vi "InputPad.vi"(10 "Increments":enum32{"0.01", "0.1", "1", "10"}(radio), 11 "Num in":sgl) -> (3 "Num out":dbl format="%6.2f")   [LabVIEW 2012, in "StimulCtrls.lvlib"]
doc: "This VI is to create a two-digit number for cohort/electrode properties, including\n1. Frequency\n2. Pulse Width\n3. Signal Amplitude"
uses:
  StimulCtrls.lvlib
  UserControl/PadEnum.ctl
panel:
  in  "Enter":bool
  in  "Backspace":bool
  in  "Clear":bool
  in  "Up":bool
  in  "Down":bool
  in  "Dot":bool
  in  "NUM 9":bool
  in  "NUM 8":bool
  in  "NUM 7":bool
  in  "NUM 6":bool
  in  "NUM 5":bool
  in  "NUM 4":bool
  in  "NUM 3":bool
  in  "NUM 2":bool
  in  "NUM 1":bool
  in  "NUM 0":bool
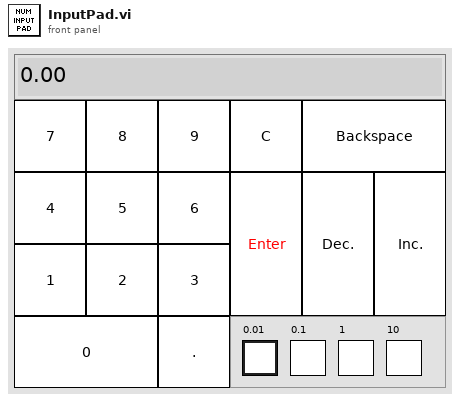
[diagram p1: front panel]
types:
  T1 = typedef "StimulCtrls.lvlib/PadEnum.ctl" = enum16{"Clear", "Inc/Dec", "Decrease", "Wait", "Exit", "Backspace", "InputDigit"}
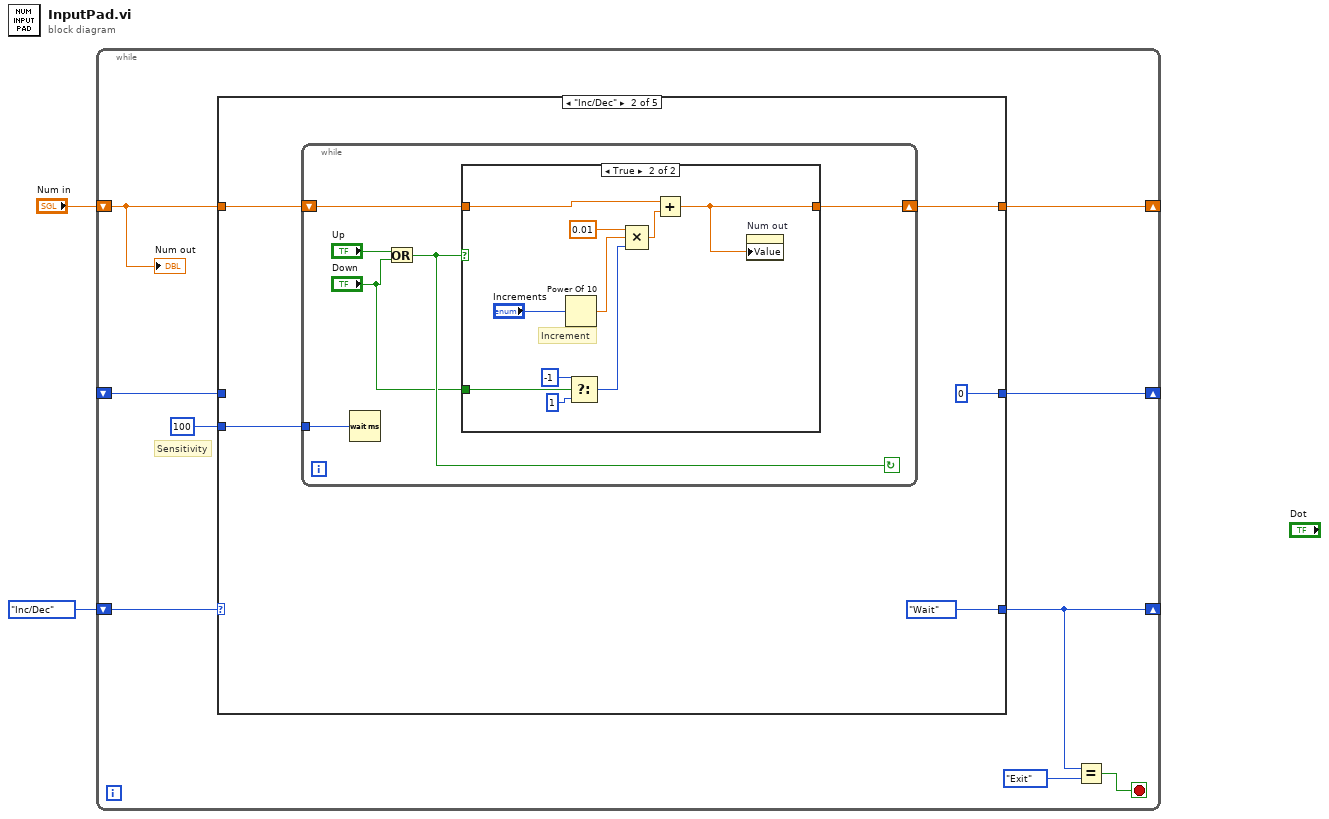
[diagram p0: block diagram]
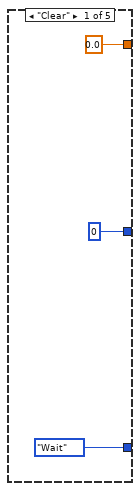
[diagram p2: hidden frame]
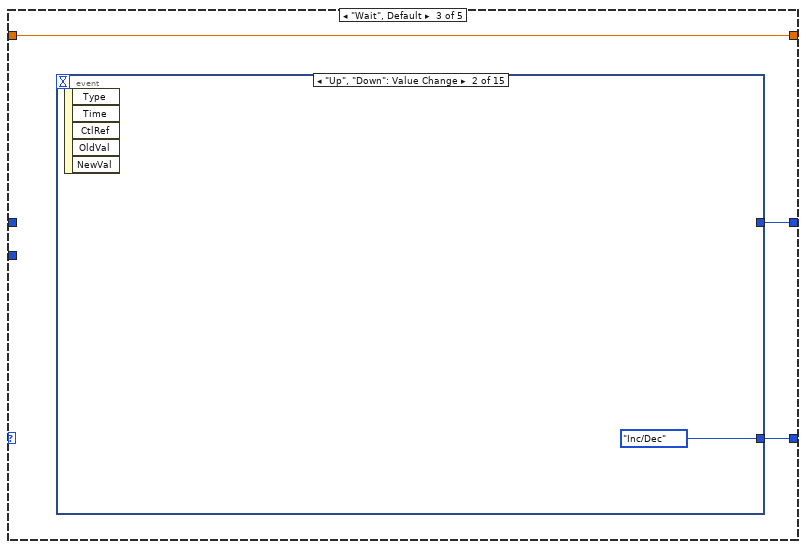
[diagram p4: hidden frame]
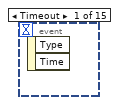
[diagram p5: hidden frame]
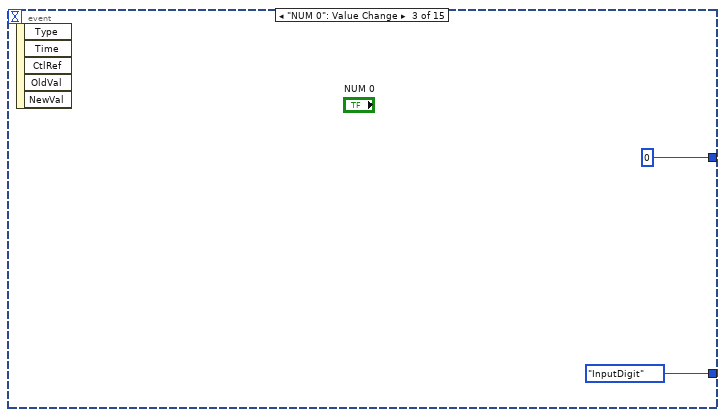
[diagram p6: hidden frame]
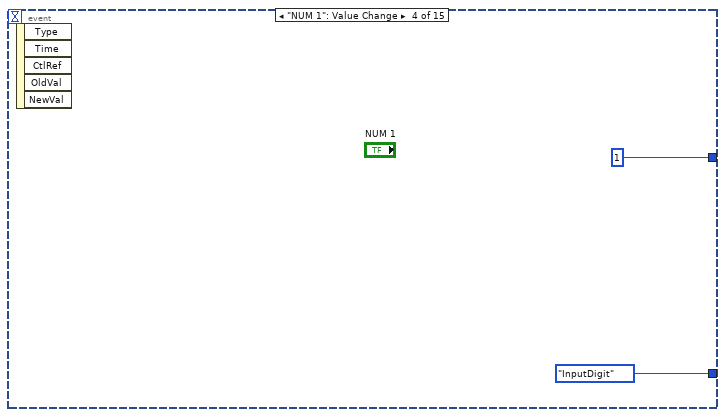
[diagram p7: hidden frame]
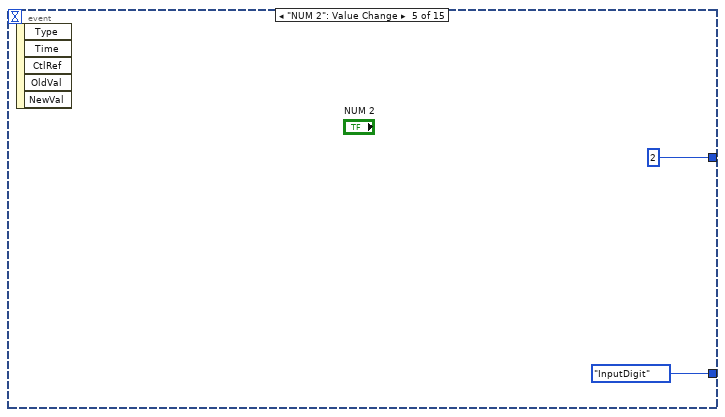
[diagram p8: hidden frame]
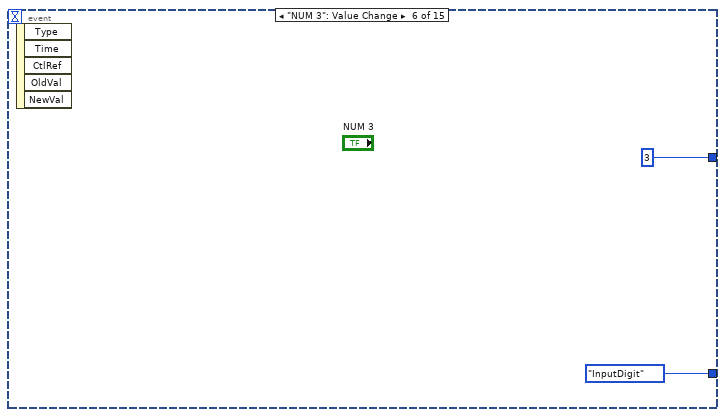
[diagram p9: hidden frame]
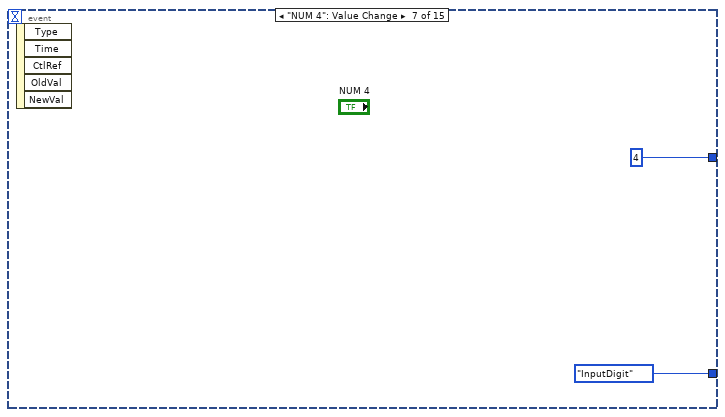
[diagram p10: hidden frame]
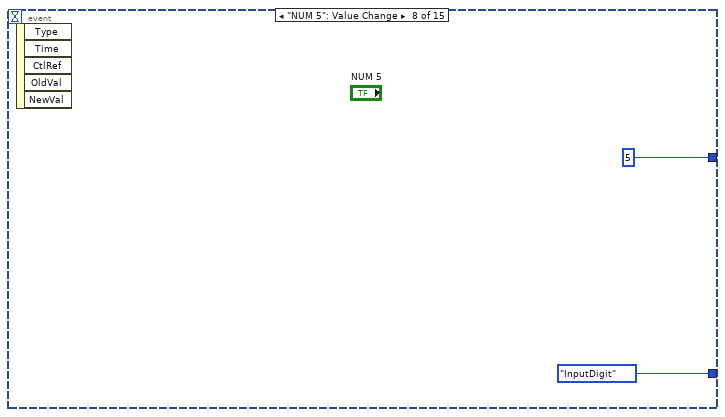
[diagram p11: hidden frame]
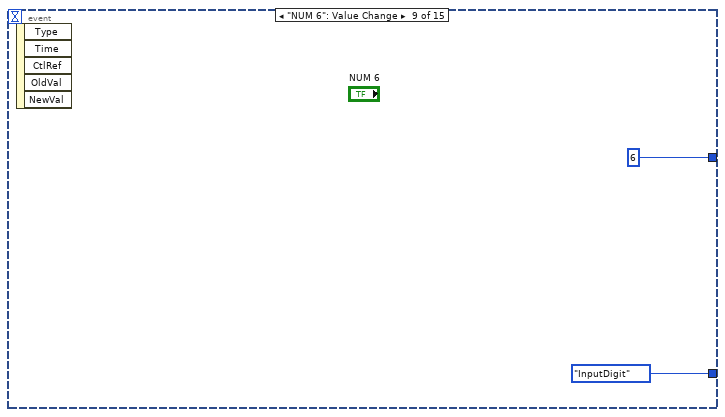
[diagram p12: hidden frame]
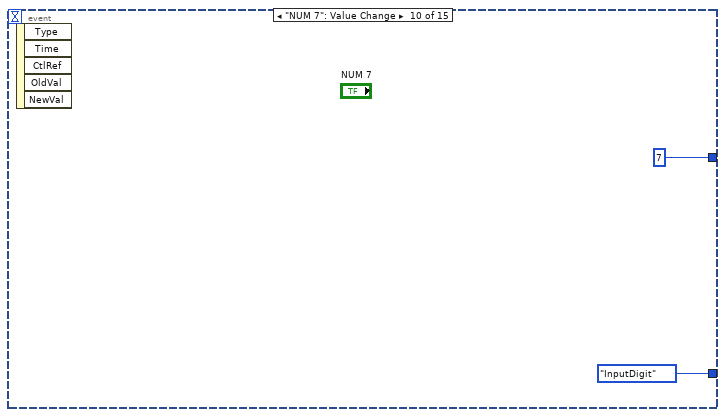
[diagram p13: hidden frame]
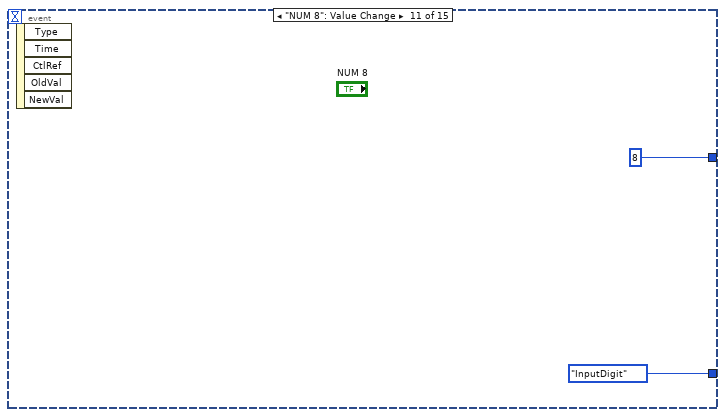
[diagram p14: hidden frame]
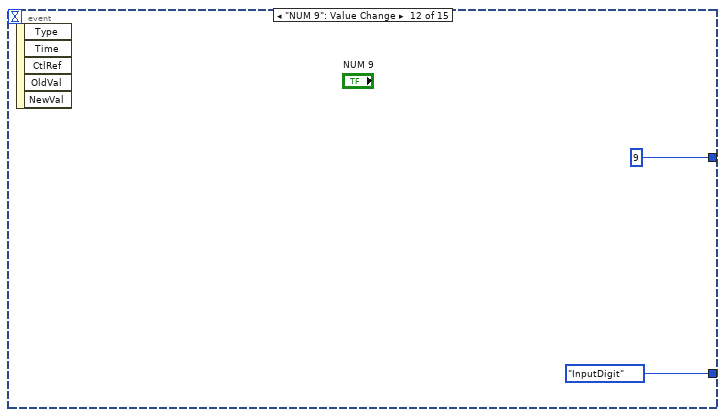
[diagram p15: hidden frame]
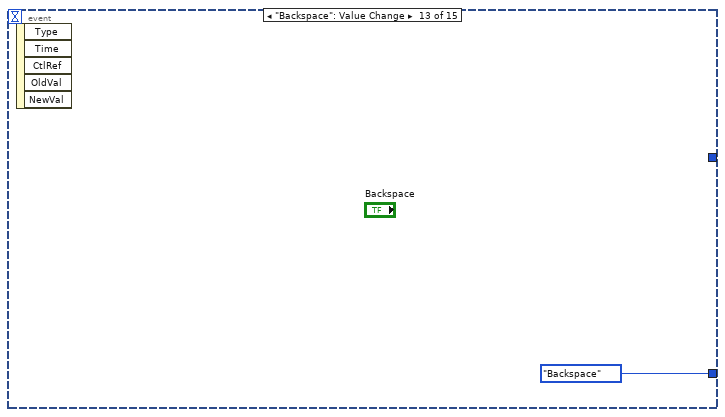
[diagram p16: hidden frame]
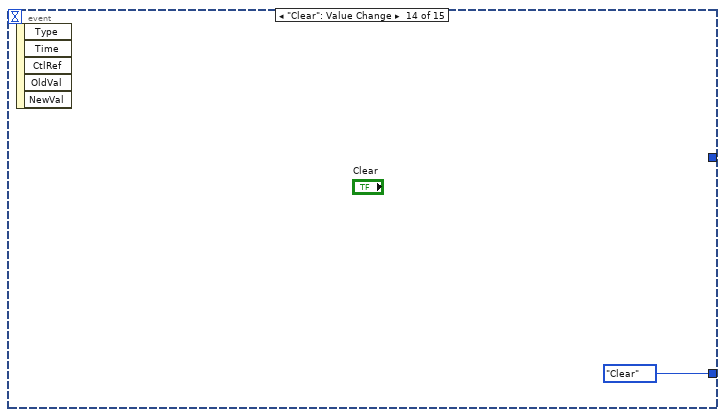
[diagram p17: hidden frame]
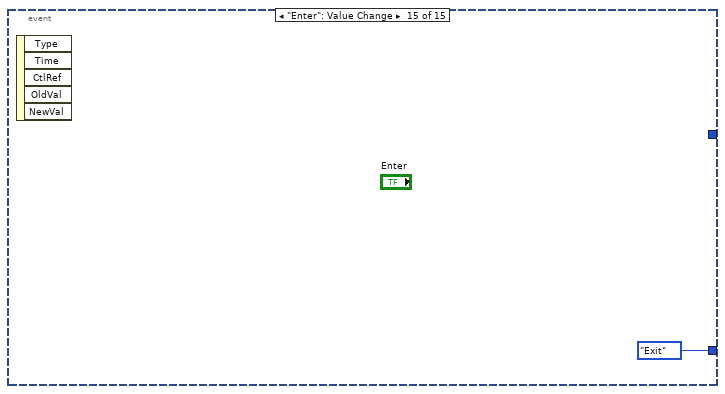
[diagram p18: hidden frame]
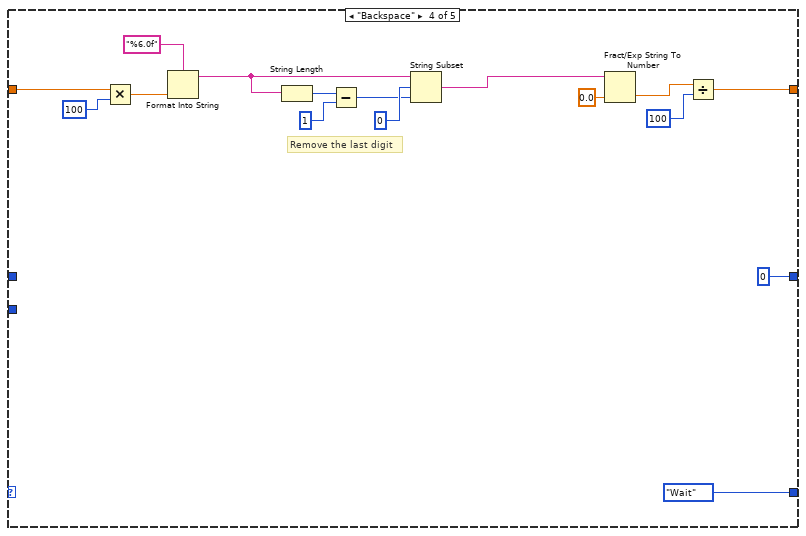
[diagram p19: hidden frame]
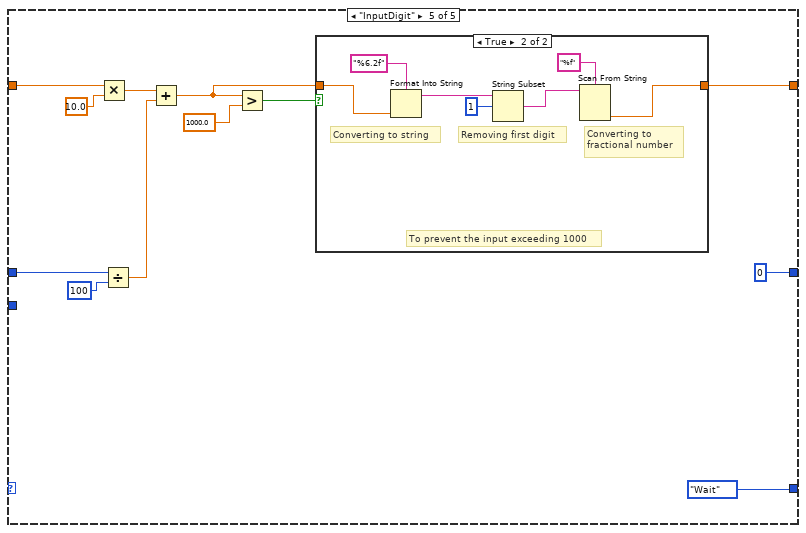
[diagram p20: hidden frame]
diagram:
  n1 = while {
    shift-right: [w7] -> _
    shift-left: PadEnum."Inc/Dec" -> [w10]
    shift-right: [w9] -> _
    shift-left: "Num in" -> [w3]
    shift-right: [w6] -> _
    shift-left: _ -> [w5]
    stop <- w11 stop-if-true
    # "Sensitivity"
    n2 = case shown="\"Inc/Dec\"" w10 {
      tunnel: [PadEnum."Wait" ("x") PadEnum."Wait" ("x") w39 PadEnum."Wait" ("x") PadEnum."Wait" ("x")] -> w7
      tunnel: [0.0 ("Num in") w18 w38 w72 w80] -> w9
      tunnel: w3 -> [_ w19 w38 w77 w91]
      tunnel: [0 0 w37 0 0] -> w6
      tunnel: w5 -> [_ _ _ _ w87]
      tunnel: u32 100 ("milliseconds to wait") -> [_ w15 _ _ _]
      frame "Clear" {
      }
      frame "Inc/Dec" {
        n3 = while {
          shift-right: [w24] -> w18
          shift-left: w19 -> [w25]
          tunnel: w15 -> [w23]
          stop <- w22 continue-if-true
          n4 = Wait (ms)(milliseconds to wait=w23) -> ()  [unwired: 1 out]
          n5 = Or(x="Up", y="Down") -> (x .or. y?=w22:bool)
          n6 = case shown="True" w22 {
            tunnel: w25 -> [w26 w36]
            tunnel: [w26 w35] -> w24
            tunnel: "Down" -> [_ w33]
            frame False {
            }
            frame True {
              # "Increment"
              n7 = Power Of 10(x="Increments") -> (10^x=w28:dbl)
              n8 = Select(t=-1, s=w33, f=1) -> (s? t:f=w27:i32)
              n9 = Compound Arithmetic op=MULTIPLY(0.01 ("y"), w28, w27) -> (w30:dbl)
              n10 = Add(x=w36, y=w30) -> (x+y=w35:dbl)
              n11 = property on="Num out" class="DigNum (strict)"("Value"=w35) -> ()  [unwired: 2 in, 2 out]
            }
          }
        }
      }
      frame "Wait", Default {
        n12 = event shown="[1] \"Up\", \"Down\": Value Change" {
          selector: _ -> [_ _ _ _ _ _ _ _ _ _ _ _ _ _ _]
          dyn-events: _ -> [_ _ _ _ _ _ _ _ _ _ _ _ _ _ _]
          timeout: _ -> [_ _ _ _ _ _ _ _ _ _ _ _ _ _ _]
          tunnel: [_ PadEnum."Inc/Dec" ("x") PadEnum."InputDigit" ("x") PadEnum."InputDigit" ("x") PadEnum."InputDigit" ("x") PadEnum."InputDigit" ("x") PadEnum."InputDigit" ("x") PadEnum."InputDigit" ("x") PadEnum."InputDigit" ("x") PadEnum."InputDigit" ("x") PadEnum."InputDigit" ("x") PadEnum."InputDigit" ("x") PadEnum."Backspace" ("x") PadEnum."Clear" ("x") PadEnum."Exit" ("x")] -> w39
          tunnel: [_ _ 0 1 2 3 4 5 6 7 8 9 _ _ _] -> w37
          event Timeout {
            n13 = event-data() -> ()  [unwired: 1 in, 2 out]
          }
          event "Up", "Down": Value Change {
            n14 = event-data() -> ()  [unwired: 1 in, 5 out]
          }
          event "NUM 0": Value Change {
            n15 = event-data() -> ()  [unwired: 1 in, 5 out]
          }
          event "NUM 1": Value Change {
            n16 = event-data() -> ()  [unwired: 1 in, 5 out]
          }
          event "NUM 2": Value Change {
            n17 = event-data() -> ()  [unwired: 1 in, 5 out]
          }
          event "NUM 3": Value Change {
            n18 = event-data() -> ()  [unwired: 1 in, 5 out]
          }
          event "NUM 4": Value Change {
            n19 = event-data() -> ()  [unwired: 1 in, 5 out]
          }
          event "NUM 5": Value Change {
            n20 = event-data() -> ()  [unwired: 1 in, 5 out]
          }
          event "NUM 6": Value Change {
            n21 = event-data() -> ()  [unwired: 1 in, 5 out]
          }
          event "NUM 7": Value Change {
            n22 = event-data() -> ()  [unwired: 1 in, 5 out]
          }
          event "NUM 8": Value Change {
            n23 = event-data() -> ()  [unwired: 1 in, 5 out]
          }
          event "NUM 9": Value Change {
            n24 = event-data() -> ()  [unwired: 1 in, 5 out]
          }
          event "Backspace": Value Change {
            n25 = event-data() -> ()  [unwired: 1 in, 5 out]
          }
          event "Clear": Value Change {
            n26 = event-data() -> ()  [unwired: 1 in, 5 out]
          }
          event "Enter": Value Change {
            n27 = event-data() -> ()  [unwired: 1 in, 5 out]
          }
        }
      }
      frame "Backspace" {
        # "Remove the last digit"
        n28 = Multiply(x=w77, y=100) -> (x*y=w73:dbl)
        n29 = Format Into String(format string="%6.0f", w73) -> (resulting string=w74:string)  [unwired: 2 in, 1 out]
        n30 = String Length(string=w74) -> (length=w68:i32)
        n31 = Subtract(x=w68, y=1) -> (x-y=w66:i32)
        n32 = String Subset(string=w74, offset (0)=0, length (rest)=w66) -> (substring=w76:string)
        n33 = Fract/Exp String To Number(string=w76, default (0 dbl)=0.0 ("default (0 DBL)")) -> (number=w71:dbl)  [unwired: 2 in, 1 out]
        n34 = Divide(x=w71, y=100) -> (x/y=w72:dbl)
      }
      frame "InputDigit" {
        n35 = Multiply(x=w91, y=10.0) -> (x*y=w89:dbl)
        n36 = Divide(x=w87, y=100) -> (x/y=w88:dbl)
        n37 = Add(x=w89, y=w88) -> (x+y=w81:dbl)
        n38 = Greater?(x=w81, y=1000.0) -> (0:w82:bool)
        n39 = case shown="True" w82 {
          tunnel: w81 -> [w92 w99]
          tunnel: [w92 w94] -> w80
          frame False {
          }
          frame True {
            # "Converting to \nfractional number"
            # "Removing first digit"
            # "Converting to string"
            # "To prevent the input exceeding 1000"
            n40 = Format Into String(format string="%6.2f", w99) -> (resulting string=w97:string)  [unwired: 2 in, 1 out]
            n41 = String Subset(string=w97, offset (0)=1) -> (substring=w95:string)  [unwired: 1 in]
            n42 = Scan From String(format string="%f", input string=w95) -> (output 1=w94:dbl)  [unwired: 3 in, 3 out]
          }
        }
      }
    }
    n43 = Equal?(x=w7, y=PadEnum."Exit" ("x")) -> (x = y?=w11:bool)
    "Num out" <- w3
  }
